vi "set RF board frequency - interlace.vi"(1 "Board 2 Frequency Limits":T1={"Minimum"=60.0, "Maximum"=90.0, "Increment"=1.0}, 2 "Board 1 Frequency Limits":T1={"Minimum"=60.0, "Maximum"=90.0, "Increment"=1.0}, 4 "error in":errorcluster, 5 "FPGA VI Reference In":T2, 6 "Board 2 Frequency 3 (MHz)":dbl, 7 "Board 1 Frequency 3 (MHz)":dbl, 8 "Board 2 Frequency 2 (MHz)":dbl, 9 "Board 2 Frequency 1 (MHz)":dbl, 10 "Board 1 Frequency 2 (MHz)":dbl, 11 "Board 1 Frequency 1  (MHz)":dbl) -> (0 "error out":errorcluster, 3 "FPGA VI Reference Out":T2)   [LabVIEW 2014]
uses:
  <vilib>/rvi/interface/nirviReadWriteControl/nirviReadWriteControl.xnode
  openfpgaref.8.6.ctl
  FPGA Bitfiles/UHR-FleezersInst_FPGATarget_UHR-FleezersCont_IqK95Pvv9lYv5.3.lvbitx
  NiFpgaLv.dll
  <vilib>/Utility/error.llb/Error Cluster From Error Code.vi
  <vilib>/rvi/errors/niLvFpgaAdjustHostInterfaceError.vi
  <vilib>/Utility/miscctls.llb/LVMinMaxIncTypeDef.ctl
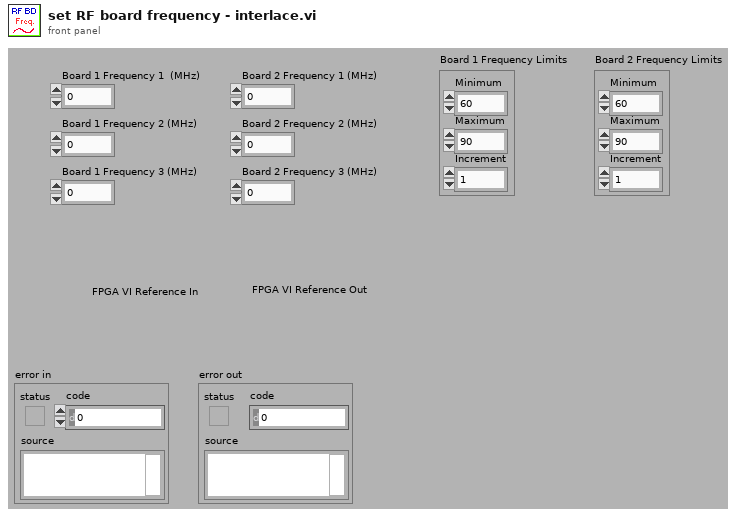
[diagram p1: front panel]
types:
  T1 = typedef "LVMinMaxIncTypeDef.ctl" = cluster{"Minimum":dbl, "Maximum":dbl, "Increment":dbl}
  T2 = typedef "openfpgaref.8.6.ctl" = refnum<k20>
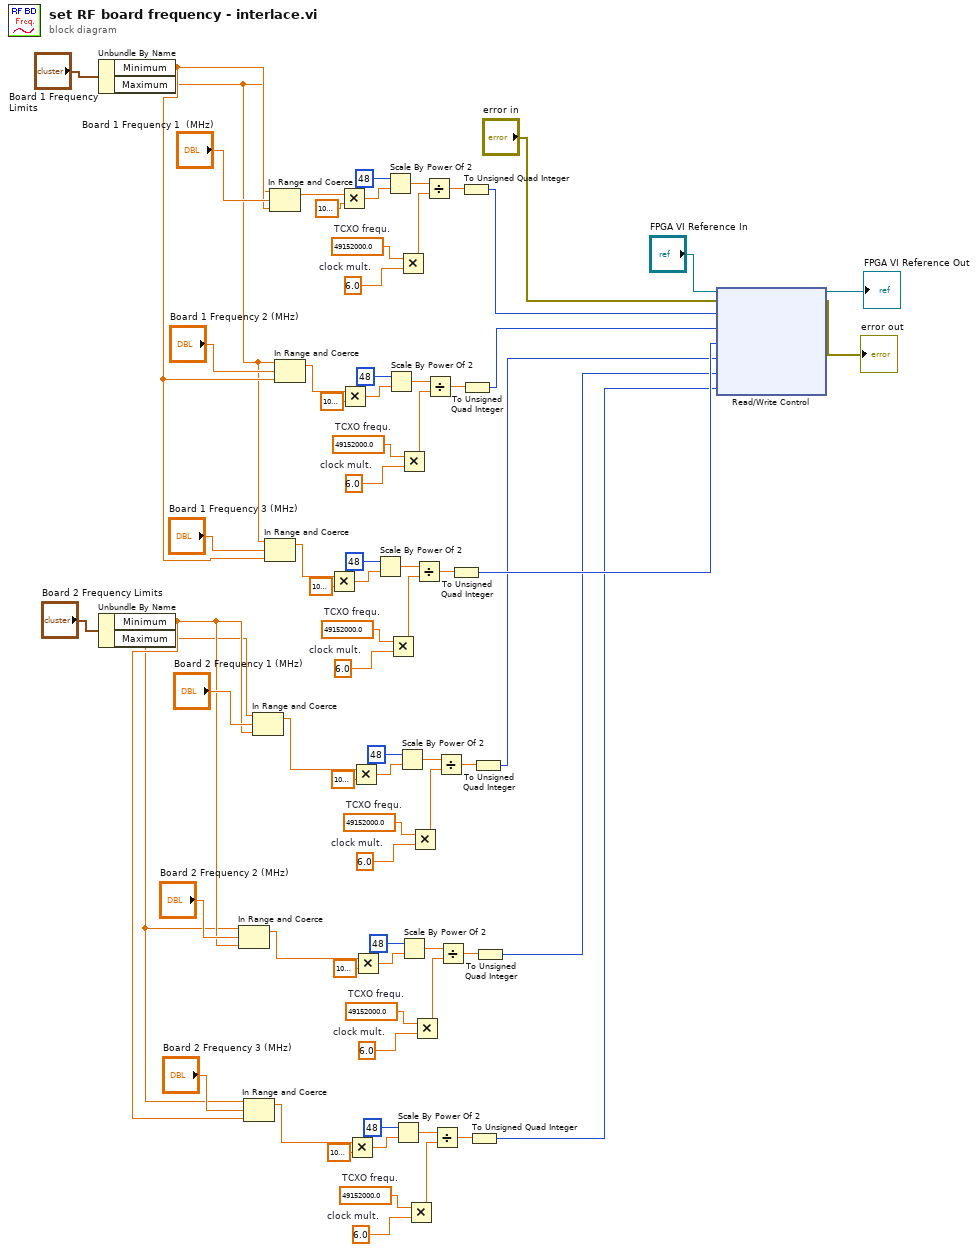
[diagram p0: block diagram]
diagram:
  w28 = 6.0  # clock mult.
  w29 = 49152000.0  # TCXO frequ.
  w36 = 6.0  # clock mult.
  w37 = 49152000.0  # TCXO frequ.
  w46 = 6.0  # clock mult.
  w47 = 49152000.0  # TCXO frequ.
  w54 = 6.0  # clock mult.
  w55 = 49152000.0  # TCXO frequ.
  w62 = 6.0  # clock mult.
  w63 = 49152000.0  # TCXO frequ.
  w70 = 6.0  # clock mult.
  w71 = 49152000.0  # TCXO frequ.
  n1 = Unbundle By Name("Board 1 Frequency Limits") -> ("Minimum"=w11:dbl, "Maximum"=w10:dbl)
  n2 = Unbundle By Name("Board 2 Frequency Limits") -> ("Minimum"=w2:dbl, "Maximum"=w1:dbl)
  n3 = In Range and Coerce(upper limit=w1, x="Board 2 Frequency 2 (MHz)", lower limit=w2) -> (coerced(x)=w5:dbl)  [unwired: 1 out]
  n4 = In Range and Coerce(upper limit=w1, x="Board 2 Frequency 3 (MHz)", lower limit=w2) -> (coerced(x)=w3:dbl)  [unwired: 1 out]
  n5 = In Range and Coerce(upper limit=w1, x="Board 2 Frequency 1 (MHz)", lower limit=w2) -> (coerced(x)=w7:dbl)  [unwired: 1 out]
  n6 = In Range and Coerce(upper limit=w10, x="Board 1 Frequency 3 (MHz)", lower limit=w11) -> (coerced(x)=w13:dbl)  [unwired: 1 out]
  n7 = In Range and Coerce(upper limit=w10, x="Board 1 Frequency 1  (MHz)", lower limit=w11) -> (coerced(x)=w17:dbl)  [unwired: 1 out]
  n8 = In Range and Coerce(upper limit=w10, x="Board 1 Frequency 2 (MHz)", lower limit=w11) -> (coerced(x)=w15:dbl)  [unwired: 1 out]
  n9 = Multiply(x=w13, y=1000000.0) -> (x*y=w39:dbl)
  n10 = Multiply(x=w17, y=1000000.0) -> (x*y=w73:dbl)
  n11 = Multiply(x=w15, y=1000000.0) -> (x*y=w65:dbl)
  n12 = Multiply(x=w3, y=1000000.0) -> (x*y=w31:dbl)
  n13 = Multiply(x=w7, y=1000000.0) -> (x*y=w57:dbl)
  n14 = Multiply(x=w5, y=1000000.0) -> (x*y=w49:dbl)
  n15 = Scale By Power Of 2(n=48, x=w39) -> (x*2^n=w41:dbl)
  n16 = Scale By Power Of 2(n=48, x=w73) -> (x*2^n=w75:dbl)
  n17 = Scale By Power Of 2(n=48, x=w65) -> (x*2^n=w67:dbl)
  n18 = Multiply(x=w37, y=w36) -> (x*y=w35:dbl)
  n19 = Scale By Power Of 2(n=48, x=w31) -> (x*2^n=w33:dbl)
  n20 = Scale By Power Of 2(n=48, x=w57) -> (x*2^n=w59:dbl)
  n21 = Multiply(x=w71, y=w70) -> (x*y=w69:dbl)
  n22 = Multiply(x=w63, y=w62) -> (x*y=w61:dbl)
  n23 = Scale By Power Of 2(n=48, x=w49) -> (x*2^n=w51:dbl)
  n24 = Multiply(x=w29, y=w28) -> (x*y=w27:dbl)
  n25 = Multiply(x=w55, y=w54) -> (x*y=w53:dbl)
  n26 = Multiply(x=w47, y=w46) -> (x*y=w45:dbl)
  n27 = Divide(x=w41, y=w35) -> (x/y=w40:dbl)
  n28 = Divide(x=w75, y=w69) -> (x/y=w74:dbl)
  n29 = Divide(x=w67, y=w61) -> (x/y=w66:dbl)
  n30 = Divide(x=w33, y=w27) -> (x/y=w32:dbl)
  n31 = Divide(x=w59, y=w53) -> (x/y=w58:dbl)
  n32 = Divide(x=w51, y=w45) -> (x/y=w50:dbl)
  n33 = To Unsigned Quad Integer(1:w40) -> (0:w24:u64)
  n34 = To Unsigned Quad Integer(1:w74) -> (0:w26:u64)
  n35 = To Unsigned Quad Integer(1:w66) -> (0:w25:u64)
  n36 = To Unsigned Quad Integer(1:w32) -> (0:w21:u64)
  n37 = To Unsigned Quad Integer(1:w58) -> (0:w23:u64)
  n38 = To Unsigned Quad Integer(1:w50) -> (0:w22:u64)
  n39 = xnode ("Read/Write Control")("FPGA VI Reference In"="FPGA VI Reference In", "error in"="error in", "BD 1 Frequency 1"=w26, "BD 1 Frequency 2"=w25, "BD 1 Frequency 3"=w24, "BD 2 Frequency 1"=w23, "BD 2 Frequency 2"=w22, "BD 2 Frequency 3"=w21) -> ("FPGA VI Reference Out"=→"FPGA VI Reference Out":T2, "error out"=→"error out":errorcluster)
